vi "Parse Error XML.vi"(9 "Code Tag Value":string, 10 "Error XML":string, 11 "AWS Core":refnum<class "IAM Session.lvclass">) -> (1 "Error Description Override":string, 2 "Error Code":i32, 3 "Warning":bool)   [LabVIEW 2015, in "NI_AWS_IAM.lvlib" / "IAM Session.lvclass"]
uses:
  IAM Session.lvclass
  Core/HTTP Request/HTTP Request.lvclass
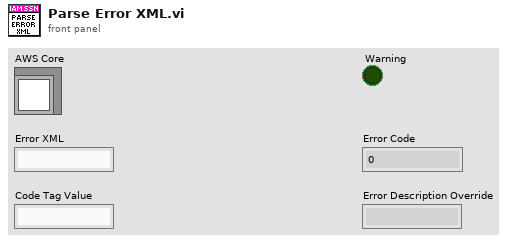
[diagram p1: front panel]
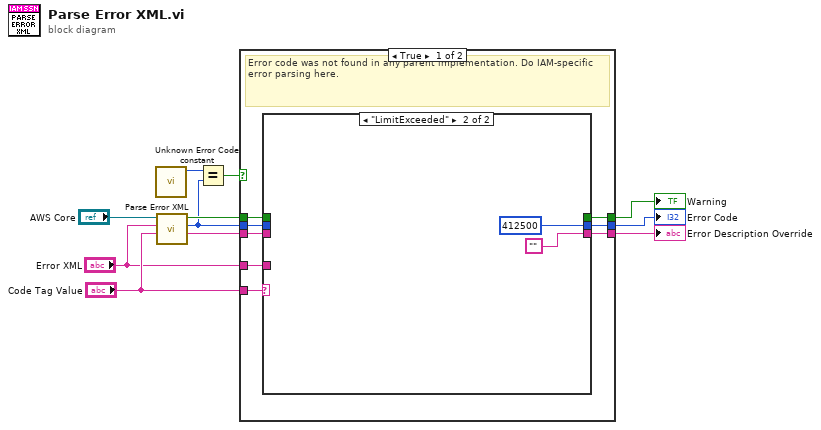
[diagram p0: block diagram]
diagram:
  n1 = call "Unknown Error Code constant.vi"() -> ("AWS Unknown Error Code value"=w11:i32)  [unwired: 11 in]
  n2 = call-parent "Parse Error XML.vi"("Code Tag Value"="Code Tag Value", "Error XML"="Error XML", "AWS Core"="AWS Core") -> ("Error Description Override"=w7:string, "Error Code"=w8:i32, "Warning"=w9:bool)  [unwired: 6 in]
  n3 = Equal?(x=w11, y=w8) -> (x = y?=w10:bool)
  n4 = case shown="True" w10 {
    tunnel: w9 -> [w17 w27]
    tunnel: w7 -> [w15 w26]
    tunnel: [w14 w27] -> w4
    tunnel: [w12 w26] -> w6
    tunnel: [w13 w25] -> w5
    tunnel: "Error XML" -> [w19 _]
    tunnel: "Code Tag Value" -> [w18 _]
    tunnel: w8 -> [w16 w25]
    frame True {
      # "Error code was not found in any parent implementation. Do IAM-specific error parsing here."
      n5 = case shown="\"LimitExceeded\"" w18 {
        tunnel: w19 -> [_ _]
        tunnel: w17 -> [w22 _]
        tunnel: w16 -> [w21 _]
        tunnel: w15 -> [w20 _]
        tunnel: [w22 _] -> w14
        tunnel: [w21 412500] -> w13
        tunnel: [w20 ""] -> w12
        frame Default {
          # "Unknown error code, use default error from parent"
        }
        frame "LimitExceeded" {
        }
      }
    }
    frame False {
      # "Parent method already assigned an error code"
    }
  }
  "Error Description Override" <- w6
  "Warning" <- w4
  "Error Code" <- w5
